vi "Get All Callers Paths.vi"(8 "错误输入（无错误）":errorcluster, 11 "VI Ref In":refnum<vi>) -> (0 "错误输出":errorcluster, 2 "Callers' Paths":path[](array[path]), 3 "VI Ref Out":refnum<vi>)   [LabVIEW 2012, in "VIRef.lvlib"]
uses:
  VIRef.lvlib
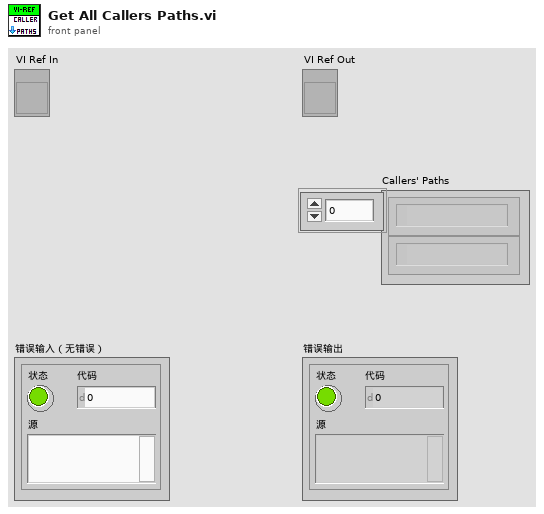
[diagram p1: front panel]
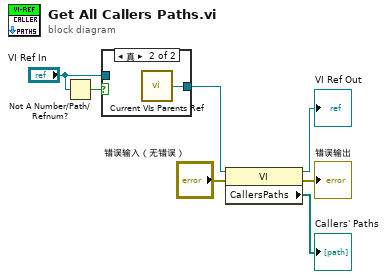
[diagram p0: block diagram]
diagram:
  n1 = Not A Number/Path/Refnum?(number/path/refnum="VI Ref In") -> (NaN/Path/Refnum?=w6:bool)
  n2 = case shown="真" w6 {
    tunnel: [w8 w9] -> w4
    tunnel: "VI Ref In" -> [w8 _]
    frame False {
    }
    frame True {
      n3 = call "Current VIs Parents Ref.vi"() -> ("Calling VI's Reference"=w9:refnum<vi>)  [unwired: 2 in]
    }
  }
  n4 = property class="VI"(reference=w4, error in="错误输入（无错误）") -> (reference out=→"VI Ref Out":refnum<vi>, error out=→"错误输出":errorcluster, "CallersPaths"=→"Callers' Paths":path[])
